vi "rotFeaBendingMode.vi"(8 "error in (no error)":errorcluster, 9 "Mirror DOF (um)":dbl[](array[numeric]), 10 "Mirror":enum16{"M1M3", "M2"}(ring), 11 "BendModeToForce in":refnum<class "BendModeToForce.lvclass">) -> (0 "error out":errorcluster, 2 "Transformed Mirror DOF (um)":dbl[](array[numeric]), 3 "BendModeToForce out":refnum<class "BendModeToForce.lvclass">)   [LabVIEW 2016, in "BendModeToForce.lvclass"]
doc: "Rotate the bending mode (degree of freedom, DOF) from Bo's FEA model to Chris's FEA model. This function should be removed in the final once there is a unified FEA model."
uses:
  BendModeToForce.lvclass
  BendModeToForce.lvclass/BendModeToForce.ctl
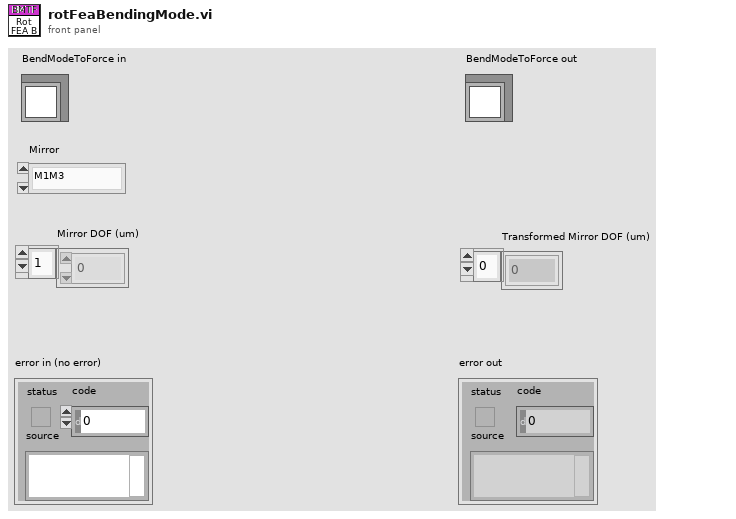
[diagram p1: front panel]
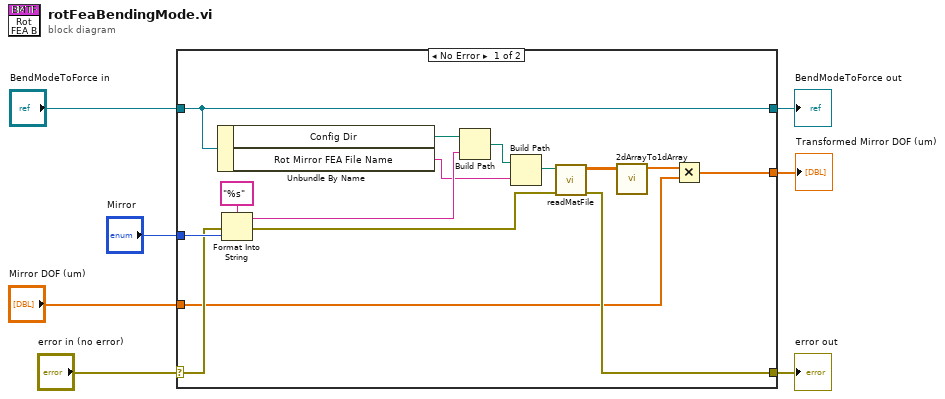
[diagram p0: block diagram]
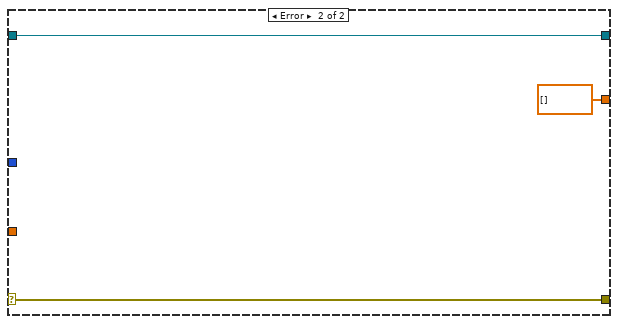
[diagram p2: hidden frame]
diagram:
  n1 = case shown="No Error" "error in (no error)" {
    selector: "error in (no error)" -> [w20 w25]
    tunnel: [w12 w25] -> w6
    tunnel: [w19 w24] -> w4
    tunnel: "BendModeToForce in" -> [w19 w24]
    tunnel: "Mirror" -> [w21 _]
    tunnel: "Mirror DOF (um)" -> [w9 _]
    tunnel: [w8 dbl[] []] -> w1
    frame No Error {
      n2 = Unbundle By Name(w19) -> ("Config Dir"=w18:path, "Rot Mirror FEA File Name"=w15:string)
      n3 = Format Into String(format string="%s", error in=w20, w21) -> (resulting string=w16:string, error out=w13:errorcluster)  [unwired: 1 in]
      n4 = Build Path(base path=w18, name or relative path=w16) -> (appended path=w17:path)
      n5 = Build Path(base path=w17, name or relative path=w15) -> (appended path=w14:path)
      n6 = call "readMatFile.vi"("error in (no error)"=w13, "Path"=w14) -> ("error out"=w12:errorcluster, "Matrix"=w11:dbl[][])  [unwired: 8 in]
      n7 = call "2dArrayTo1dArray.vi"("2D Array"=w11) -> ("1D Array"=w10:dbl[])  [unwired: 10 in]
      n8 = Multiply(x=w10, y=w9) -> (x*y=w8:dbl[])
    }
    frame Error {
    }
  }
  "error out" <- w6
  "BendModeToForce out" <- w4
  "Transformed Mirror DOF (um)" <- w1
